vi "Temp Messzelle.vi"() -> (3 "Temp. Messzelle":i32)   [LabVIEW 2020, in "EPA 1065.lvlib" / "HovaCAL Interference verificaton.lvlib"]
uses:
  HovaCAL Interference verificaton.lvlib
  Allgemein/allgemeine Sub-VIs.lvlib
  Seiten/FT-IR/Algebraic Modul/Algebraic Modul.lvlib
  Seiten/FT-IR/Algebraic Modul/FGV Algebraic Aktionen.ctl
  Sprachverwaltung/Sprachverwaltung.lvlib
  Sprachverwaltung/FGV Aktion Tabelle zerlegen.ctl
  Seiten/FT-IR/FT-IR.lvlib
  Seiten/FT-IR/FGV FT-IR Gasliste Aktionen.ctl
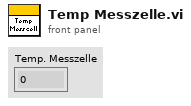
[diagram p1: front panel]
types:
  T1 = typedef "FT-IR.lvlib/FGV FT-IR Gasliste Aktionen.ctl" = enum16{"lesen", "Gasliste FT-IR", "Gasliste ausgelesen", "laden", "speichern", "löschen"}
  T2 = typedef "Sprachverwaltung.lvlib/FGV Aktion Tabelle zerlegen.ctl" = enum16{"laden", "vereinzeln", "speichern"}
  T3 = typedef "FT-IR.lvlib/Algebraic Modul.lvlib/FGV Algebraic Aktionen.ctl" = enum16{"lesen", "laden", "speichern", "berechnen", "schreiben"}
  T4 = typedef "String - Ausgabefeld.ctl" = string
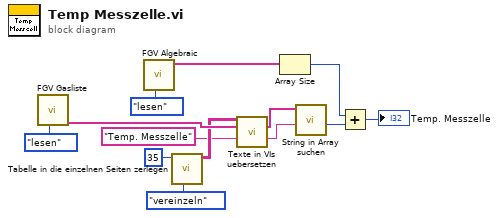
[diagram p0: block diagram]
diagram:
  n1 = call "FGV Gasliste.vi"("Aktionen"=FGV_FT-IR_Gasliste_Aktionen."lesen") -> ("Aktuelle Gasliste gesamt"=w10:T4[])  [unwired: 8 in, 2 out]
  n2 = call "FGV Algebraic.vi"("Aktionen Algebraic"=FGV_Algebraic_Aktionen."lesen") -> ("Namen"=w9:string[])  [unwired: 6 in, 4 out]
  n3 = call "Tabelle in die einzelnen Seiten zerlegen.vi"("Aktion"=FGV_Aktion_Tabelle_zerlegen."vereinzeln", "Index (Seite)"=35) -> ("Sprachliste"=w8:string[][])  [unwired: 7 in, 2 out]
  n4 = call "Texte in VIs uebersetzen.vi"("Sprachliste"=w8, "String-Array zum Übersetzen"=w10, "String zum Übersetzen"="Temp. Messzelle" ("Neues Element/Teil-Array")) -> ("String-Array zum Übersetzen"=w11:string[], "String zum Übersetzen"=w6:string)  [unwired: 8 in, 3 out]
  n5 = Array Size(array=w9) -> (size(s)=w4:i32)
  n6 = call "String in Array suchen.vi"("Nach String/Zeichen suchen (-)"=w6, "String-Array"=w11) -> ("Index"=w2:i32)  [unwired: 7 in, 2 out]
  n7 = Add(x=w4, y=w2) -> (x+y=→"Temp. Messzelle":i32)
